vi "SmartSEM Remote API detectors.vi"(7 "Iterations":u32=3, 8 "error in":errorcluster, 9 "Det B Type":string, 10 "Det A Type":string, 11 "ActiveX Container":refnum<k7>(container)) -> (0 "error out":errorcluster, 3 "reference out":refnum<k7>)   [LabVIEW 2018]
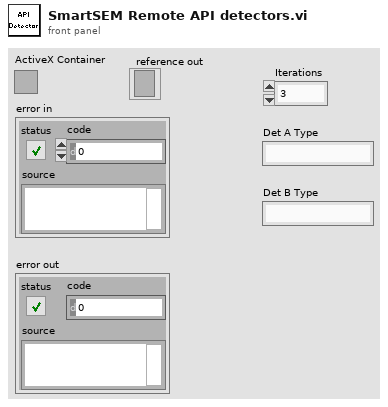
[diagram p1: front panel]
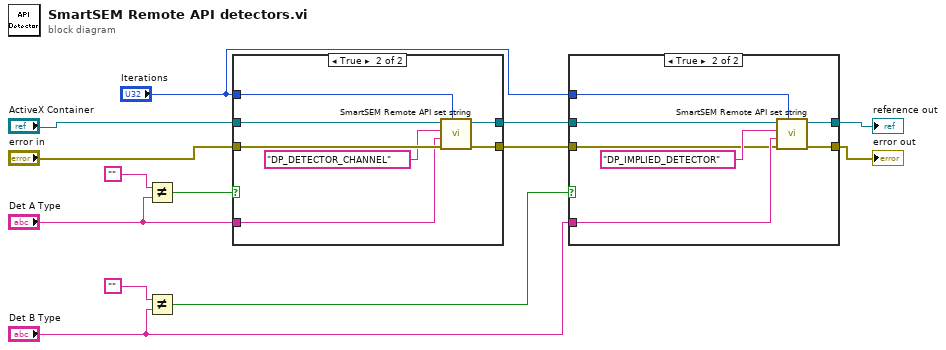
[diagram p0: block diagram]
diagram:
  n1 = Not Equal?(x="", y="Det A Type") -> (x != y?=w11:bool)
  n2 = Not Equal?(x="", y="Det B Type") -> (x != y?=w7:bool)
  n3 = case shown="True" w11 {
    tunnel: "ActiveX Container" -> [w15 w22]
    tunnel: "error in" -> [w14 w21]
    tunnel: "Det A Type" -> [_ w20]
    tunnel: [w15 w17] -> w4
    tunnel: [w14 w16] -> w5
    tunnel: "Iterations" -> [_ w18]
    frame False {
    }
    frame True {
      n4 = call "SmartSEM Remote API set string.vi"("Iterations"=w18, "error in"=w21, "vValue"=w20, "lpszParam"="DP_DETECTOR_CHANNEL" ("lpszCommand"), "ActiveX Container"=w22) -> ("error out"=w16:errorcluster, "reference out"=w17:refnum<k7>)  [unwired: 5 in]
    }
  }
  n5 = case shown="True" w7 {
    tunnel: w4 -> [w24 w26]
    tunnel: w5 -> [w23 w25]
    tunnel: "Det B Type" -> [_ w31]
    tunnel: [w24 w29] -> w1
    tunnel: [w23 w28] -> w3
    tunnel: "Iterations" -> [_ w30]
    frame False {
    }
    frame True {
      n6 = call "SmartSEM Remote API set string.vi"("Iterations"=w30, "error in"=w25, "vValue"=w31, "lpszParam"="DP_IMPLIED_DETECTOR" ("lpszCommand"), "ActiveX Container"=w26) -> ("error out"=w28:errorcluster, "reference out"=w29:refnum<k7>)  [unwired: 5 in]
    }
  }
  "error out" <- w3
  "reference out" <- w1
